vi "Get Test Channel Move In Next.vi"(8 "error in (no error)":errorcluster, 11 "Abstract Test Channel Move In Next Msg in":refnum<class "Abstract Test Channel Move In Next Msg.lvclass">) -> (0 "error out":errorcluster, 2 "Test Channel Move In Next":bool, 3 "Abstract Test Channel Move In Next Msg out":refnum<class "Abstract Test Channel Move In Next Msg.lvclass">)   [LabVIEW 2013, in "Test Channel Model.lvlib" / "Abstract Test Channel Move In Next Msg.lvclass"]
uses:
  Abstract Test Channel Move In Next Msg.lvclass
  Abstract Test Channel Move In Next Msg.lvclass/Abstract Test Channel Move In Next Msg.ctl
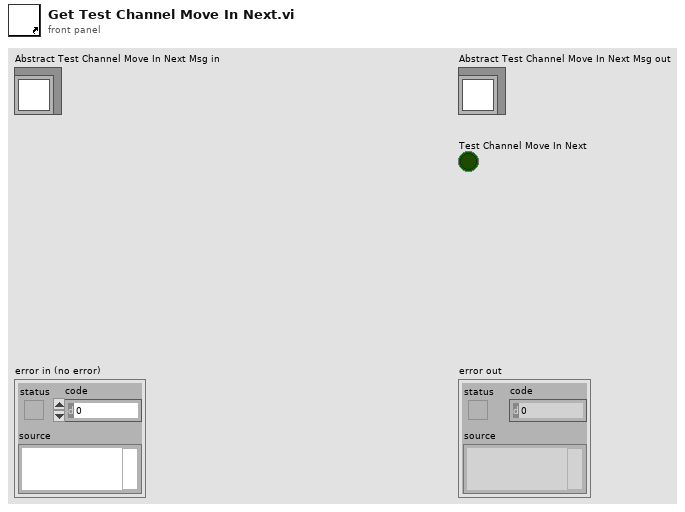
[diagram p1: front panel]
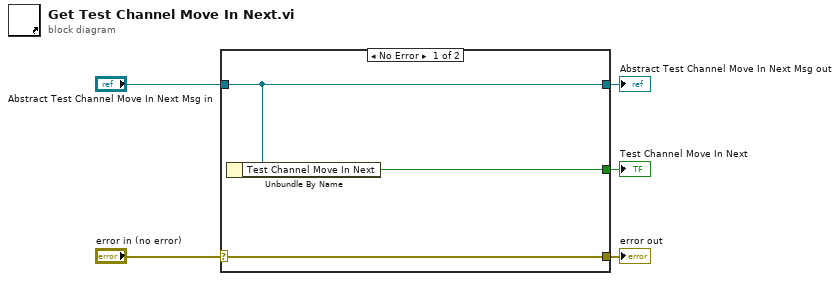
[diagram p0: block diagram]
diagram:
  n1 = case shown="No Error" "error in (no error)" {
    selector: "error in (no error)" -> [w8 w9]
    tunnel: [w8 w9] -> w4
    tunnel: [w7 w10] -> w2
    tunnel: "Abstract Test Channel Move In Next Msg in" -> [w7 w10]
    tunnel: [w6 _] -> w1
    frame No Error {
      n2 = Unbundle By Name(w7) -> ("Test Channel Move In Next"=w6:bool)
    }
    frame Error {
    }
  }
  "error out" <- w4
  "Abstract Test Channel Move In Next Msg out" <- w2
  "Test Channel Move In Next" <- w1
